vi "Connect.vi"(6 "error in":errorcluster, 7 "Address":string, 9 "Websocket Handler in":refnum<class "Websocket Handler.lvclass">) -> (0 "error out":errorcluster, 3 "Websocket Handler out":refnum<class "Websocket Handler.lvclass">)   [LabVIEW 2020, in "wamplv.lvlib" / "Websocket Handler.lvclass"]
uses:
  Websocket Handler.lvclass
  C:/local/wamplv/Private/Comm Handlers/CommHandlerBase/CommHandlerBase.lvclass
  Websocket Handler.lvclass/Websocket Handler.ctl
  <vilib>/MediaMongrels Ltd/WebSockets/WebSockets/WebSocket Client/WebSocket Client.lvclass
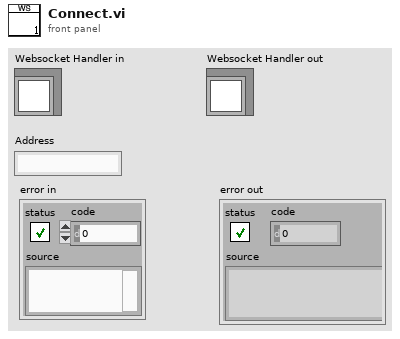
[diagram p1: front panel]
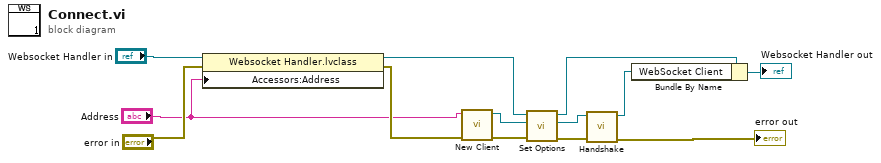
[diagram p0: block diagram]
diagram:
  n1 = property class="Websocket Handler.lvclass"(reference="Websocket Handler in", error in="error in", "Accessors:Address"="Address") -> (reference out=w2:refnum<class "Websocket Handler.lvclass">, error out=w8:errorcluster)
  n2 = call <vilib>:"New Client.vi"("error in (no error)"=w8, "WebSocket URL"="Address") -> ("error out"=w5:errorcluster, "WebSocket Client out"=w6:refnum<class "WebSocket Client.lvclass">)  [unwired: 8 in]
  n3 = call "Set Options.vi"("error in"=w5, "WebSocket reference"=w6, "Websocket Handler in"=w2) -> ("error out"=w4:errorcluster, "reference out"=w3:refnum<class "WebSocket Client.lvclass">, "Websocket Handler out"=w1:refnum<class "Websocket Handler.lvclass">)  [unwired: 6 in]
  n4 = call-dynamic "Handshake.vi"("error in (no error)"=w4, "WebSocket Client in"=w3) -> ("error out"=→"error out":errorcluster, "WebSocket Client out"=w11:refnum<class "WebSocket Client.lvclass">)  [unwired: 8 in]
  n5 = Bundle By Name(cluster=w1, "WebSocket Client"=w11) -> (→"Websocket Handler out":refnum<class "Websocket Handler.lvclass">)
